vi "shuffle_seq.vi"(1 "Shuffle":bool=TRUE, 2 "Array IN":T1[](array[typedef])) -> (0 "Array OUT":T1[](array[typedef]))   [LabVIEW 2015, in "oskar_tools.lvlib"]
uses:
  oskar_tools.lvlib
  seq_line.ctl
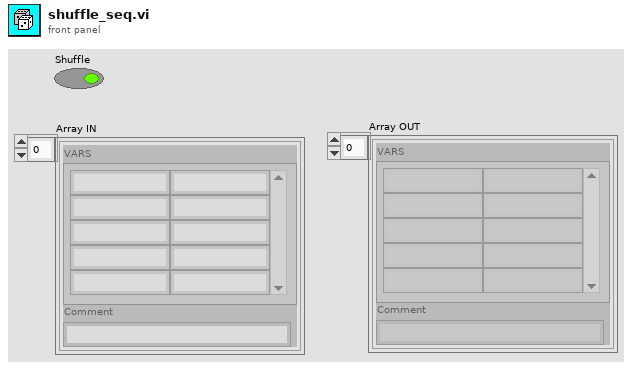
[diagram p1: front panel]
types:
  T1 = typedef "oskar_tools.lvlib/seq_line.ctl" = cluster{"VARS":string[][], "Comment":string}
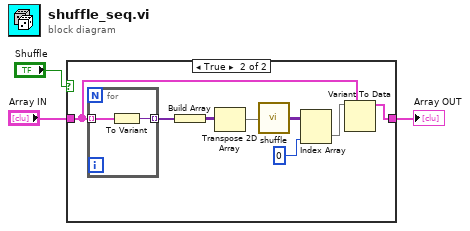
[diagram p0: block diagram]
diagram:
  n1 = case shown="True" "Shuffle" {
    tunnel: "Array IN" -> [w4 w12]
    tunnel: [w4 w11] -> w2
    frame False {
    }
    frame True {
      n2 = for {
        tunnel: w12 -> [w14] mode=indexing
        tunnel: [w13] -> w10 mode=indexing
        n3 = To Variant(anything=w14) -> (Variant=w13:variant)
      }
      n4 = Build Array(w10) -> (w7:variant[][])
      n5 = Transpose 2D Array(2D array=w7) -> (transposed array=w6:variant[][])
      n6 = call "shuffle.vi"("Array IN"=w6) -> ("Array OUT"=w9:variant[][])
      n7 = Index Array(array=w9, index (col)=0 ("disabled index (col)")) -> (element=w8:variant[])  [unwired: 1 in]
      n8 = Variant To Data(type=w12, Variant=w8) -> (data=w11:T1[])  [unwired: 1 in, 1 out]
    }
  }
  "Array OUT" <- w2
